vi "Send Rx Command.vi"(8 "error in (no error)":errorcluster, 9 "timeout in ms (0)":i32 format="%d ms", 10 "Rx Parameters":T1, 11 "Dispatcher Interface in":refnum<class "Dispatcher Interface.lvclass">) -> (0 "error out":errorcluster, 1 "timed out?":bool, 3 "Dispatcher Interface out":refnum<class "Dispatcher Interface.lvclass">)   [LabVIEW 2017, in "DSF Core.lvlib" / "Dispatcher Interface.lvclass"]
uses:
  Dispatcher Interface.lvclass
  C:/Git/DSF/Data Sharing Framework/Source/Core/Engine/Classes/Interfaces/Interface/Interface.lvclass
  Rx Parameters.ctl
  Command Data.ctl
  Command.ctl
  Parameters.ctl
  Interface/Interface.lvclass/Interface.ctl
  Debug/FIFO Flags/FIFO Flags.lvclass/FIFO Flags.ctl
  Write Dispatcher Command.vi
  Interface/Write Command.vi
  Interface/Get Command FIFO.vi
  Interface/Write RT FIFO(16B).vi
  Interface/Get Debug Flags.vi
  Debug/FIFO Flags/Get Infinite Timeouts.vi
  Interface/Errors.vi
  Interface/Command Timeout.vi
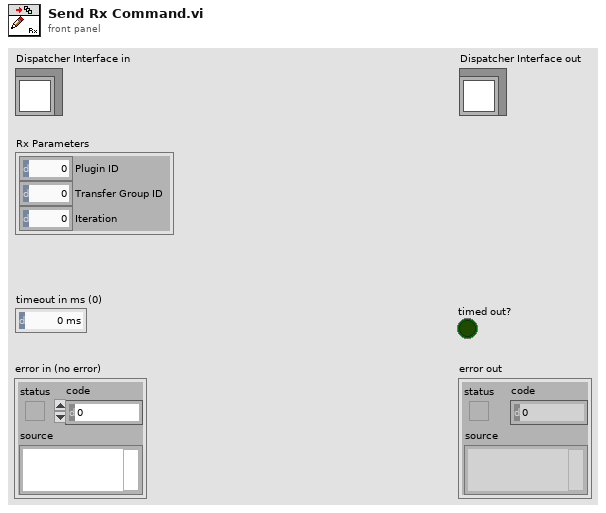
[diagram p1: front panel]
types:
  T1 = typedef "DSF Core.lvlib/Dispatcher Interface.lvclass/Rx Parameters.ctl" = cluster{"Plugin ID":i32, "Transfer Group ID":i32, "Iteration":u64}
  T2 = typedef "DSF Core.lvlib/Dispatcher Interface.lvclass/Command.ctl" = enum8{"Rx", "Tx", "Shutdown"}
  T3 = typedef "DSF Core.lvlib/Dispatcher Interface.lvclass/Parameters.ctl" = cluster{"arg1":u64, "arg2":u64}
  T4 = typedef "DSF Core.lvlib/Dispatcher Interface.lvclass/Command Data.ctl" = cluster{"Command":T2, "Parameters":T3}
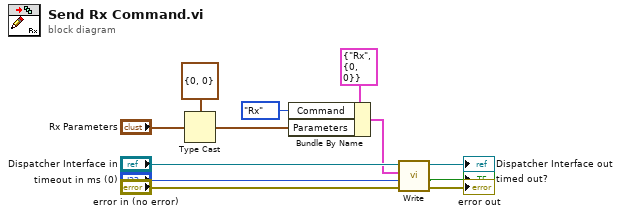
[diagram p0: block diagram]
diagram:
  n1 = Type Cast(type=T3 {"arg1"=0, "arg2"=0} ("Parameters"), x="Rx Parameters") -> (*(type *) &x=w4:T3)
  n2 = Bundle By Name(cluster=T4 {"Command"=enum."Rx", "Parameters"={"arg1"=0, "arg2"=0}} ("command"), "Command"=Command."Rx", "Parameters"=w4) -> (w2:T4)
  n3 = call-poly "Write.vi"("error in (no error)"="error in (no error)", "timeout in ms (0)"="timeout in ms (0)", "command"=w2, "Dispatcher Interface in"="Dispatcher Interface in") -> ("error out"=→"error out":errorcluster, "timed out?"=→"timed out?":bool, "Dispatcher Interface out"=→"Dispatcher Interface out":refnum<class "Dispatcher Interface.lvclass">)  [unwired: 5 in]
